vi "bbb.vi"(8 "error in (no error)":errorcluster, 11 "CBar in":refnum<class "CBar.lvclass">) -> (0 "error out":errorcluster, 3 "CBar out":refnum<class "CBar.lvclass">)   [LabVIEW 2024, in "CBar.lvclass"]
uses:
  CBar.lvclass
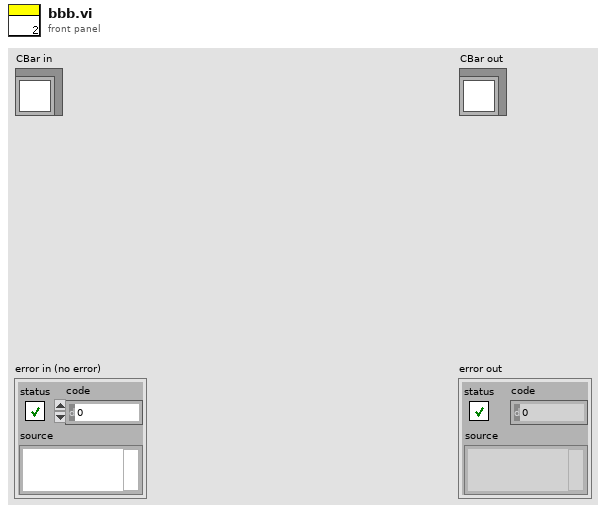
[diagram p1: front panel]
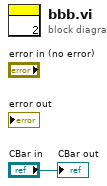
[diagram p0: block diagram]
diagram:
  "CBar out" <- "CBar in"
